vi "UV_Ctrl mode.vi"(7 "R/W (F:read)":bool, 8 "error in (no error)":errorcluster, 10 "Mode":T1 items=["MANU", "AUTO", "MANUPRO", "AUTOPRO"], 11 "VISA resource":refnum<visa-resource-name>) -> (0 "error out":errorcluster, 2 "mode":u8, 3 "VISA resource out":refnum<visa-resource-name>, 5 "Err?":bool)   [LabVIEW 8.6]
uses:
  TypeDef/UVLed_func.ctl
  TypeDef/UVLed_mode.ctl
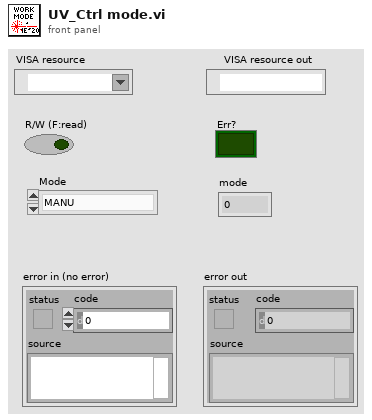
[diagram p1: front panel]
types:
  T1 = typedef "UVLed_mode.ctl" = u16
  T2 = typedef "UVLed_func.ctl" = u16
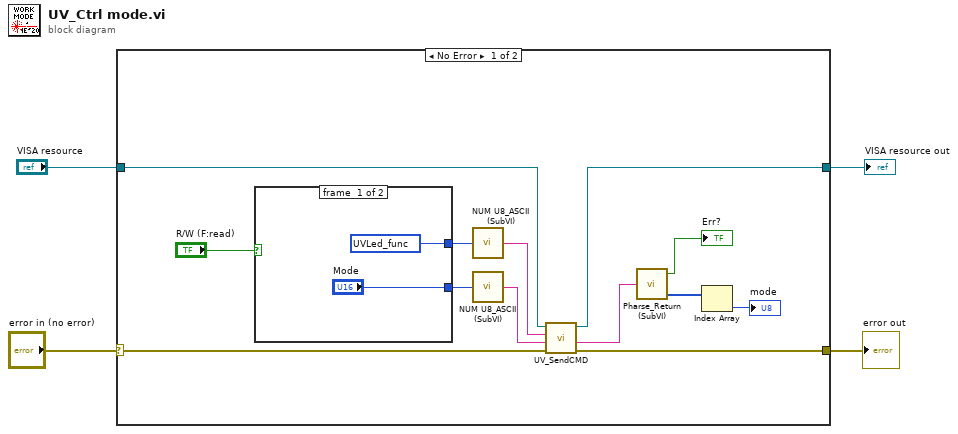
[diagram p0: block diagram]
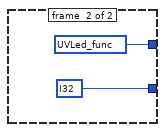
[diagram p2: hidden frame]
diagram:
  n1 = case shown="No Error" "error in (no error)" {
    selector: "error in (no error)" -> [w13 w23]
    tunnel: [w11 w23] -> w3
    tunnel: "VISA resource" -> [w14 w22]
    tunnel: [w9 w22] -> w1
    frame #0 {
      n2 = case shown="False" "R/W (F:read)" {
        tunnel: [w19 w21] -> w17
        tunnel: ["Mode" i32 ?] -> w15
        frame #0 {
          w19 = T2 ? items=["GetAllStatus", "LightOn", "LightOff", "AllForceOff", "GetMenuChnPara", "SetMenuChnPara", "GetAutoChnPara", "SetAutoChnPara", "GetMenuTemplate", "SetMenuTemplate", "GetAutoTemplate", "SetAutoTemplate", "GetTemplatePara", "SetTemplatePara", "GetMode", "SetMode", "ChkErr"] ("Function")
        }
        frame #1 {
          w21 = T2 ? items=["GetAllStatus", "LightOn", "LightOff", "AllForceOff", "GetMenuChnPara", "SetMenuChnPara", "GetAutoChnPara", "SetAutoChnPara", "GetMenuTemplate", "SetMenuTemplate", "GetAutoTemplate", "SetAutoTemplate", "GetTemplatePara", "SetTemplatePara", "GetMode", "SetMode", "ChkErr"] ("Function")
        }
      }
      n3 = call "NUM U8_ASCII (SubVI).vi"("Numeric"=w17) -> ("String out"=w16:string)
      n4 = call "NUM U8_ASCII (SubVI).vi"("Numeric"=w15) -> ("String out"=w12:string)
      n5 = call "UV_SendCMD.vi"("error in"=w13, "value"=w12, "function"=w16, "VISA resource name"=w14) -> ("error out"=w11:errorcluster, "response"=w10:string, "VISA resource name out"=w9:refnum<visa-resource-name>)  [unwired: 5 in]
      n6 = call "Pharse_Return (SubVI).vi"("buffer in"=w10) -> ("byte array"=w6:u8[], "Err?"=→"Err?":bool)  [unwired: 2 in, 1 out]
      n7 = Index Array(array=w6) -> (element=→"mode":u8)  [unwired: 1 in]
    }
    frame #1 {
    }
  }
  "error out" <- w3
  "VISA resource out" <- w1
